vi "985x-fpga-main.vi"   [LabVIEW 2020]
uses:
  <vilib>/rvi/Emulation/niFpgaGetClockAttributes.vi
  <vilib>/rvi/Emulation/niFpgaSctlEmulationGetInTimedLoop.vi
  <vilib>/rvi/Emulation/niFpgaEmulationReportErrorSimple.vi
  <vilib>/rvi/interface/RandomDataEmulation/nirviRandomDataMultiElementFPGAFIFO.vi
  <instcachedir>/0/nirviRandomDataMultiElementFPGAFIFO_3E9965BA1FAD4E7B8DABA31768A09B1F.lvgen/nirviRandomDataMultiElementFPGAFIFO_3E9965BA1FAD4E7B8DABA31768A09B1F_001.vi
  <vilib>/rvi/interface/RandomDataEmulation/niFpgaRandomDataHandleErrors.vi
  <vilib>/rvi/eio/common/nirviEmuTemplateMethod_errors.vi
  <vilib>/rvi/Emulation/niFpgaCriticalErrorInLSC.vi
  <vilib>/rvi/DataTransferAndStorage/Container/XNode/niFpgaContainer.xnode
  <vilib>/rvi/interface/RandomDataEmulation/nirviRandomDataFpgaMultiElementTemplate.vi
  <vilib>/eio/EIONode/EIONode.xnode
  <vilib>/LabVIEW Targets/FPGA/RIO/nicrio_985x_controls.llb/CAN_IO_Frame Array U32.ctl
types:
  T1 = typedef "CAN_IO_Frame Array U32.ctl" = u32[]
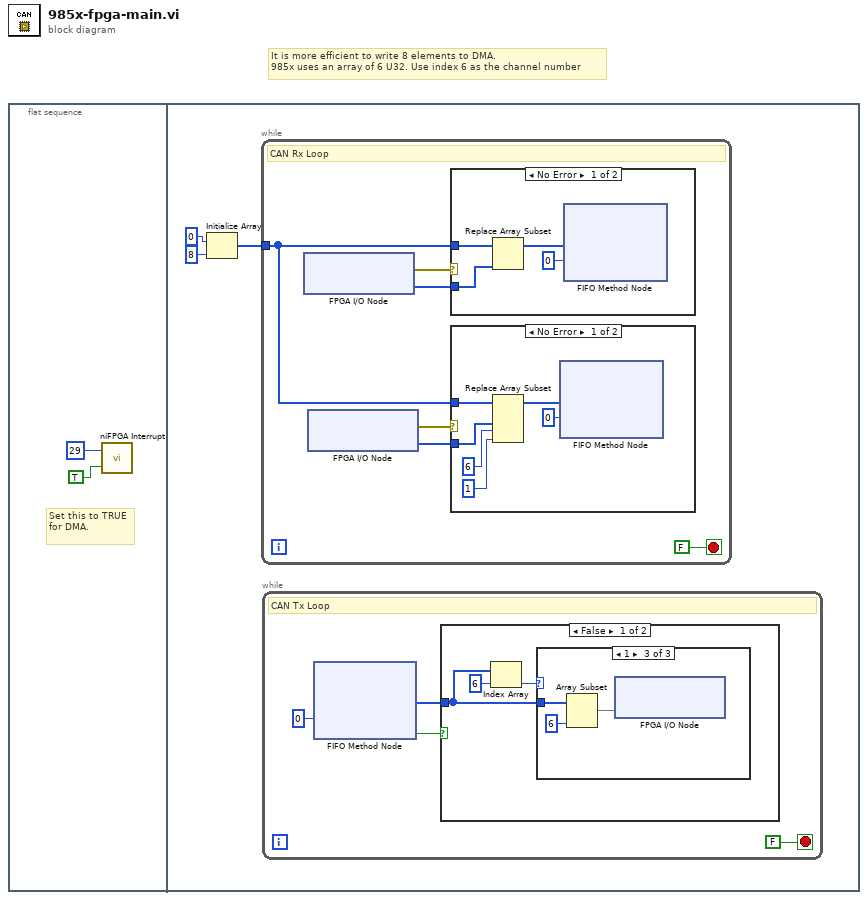
[diagram p0: block diagram]
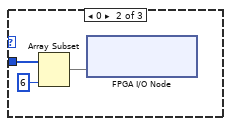
[diagram p3: hidden frame]
diagram:
  # "It is more efficient to write 8 elements to DMA.\n985x uses an array of 6 U32. Use index 6 as the channel number"
  n1 = flat-sequence {
    frame #0 {
      # "Set this to TRUE for DMA."
      n2 = call <vilib>:"niFPGA Interrupt.vi"("Wait Until Cleared (F)"=TRUE, "IRQ Number (0)"=u8 29) -> ()  [unwired: 1 in]
    }
    frame #1 {
      n3 = Initialize Array(u32 0, 8 ("dimension size")) -> (w3:u32[])
      n4 = while {
        tunnel: w3 -> [w20]
        stop <- FALSE stop-if-true
        # "CAN Rx Loop"
        n5 = xnode "FPGA I/O Node"() -> ("error out"=w24:errorcluster, "Mod8/CAN0"=w23:T1)  [unwired: 2 in, 1 out]
        n6 = xnode "FPGA I/O Node"() -> ("error out"=w22:errorcluster, "Mod8/CAN1"=w21:T1)  [unwired: 2 in, 1 out]
        n7 = case shown="No Error" w24 {
          tunnel: w20 -> [w28 _]
          tunnel: w23 -> [w27 _]
          frame No Error {
            n8 = Replace Array Subset(array=w28, new element=w27) -> (w26:u32[])  [unwired: 1 in]
            n9 = xnode ("FIFO Method Node")("Element"=w26, "Timeout"=0) -> ()  [unwired: 1 in, 2 out]
          }
          frame Error {
          }
        }
        n10 = case shown="No Error" w22 {
          tunnel: w20 -> [w34 _]
          tunnel: w21 -> [w33 _]
          frame No Error {
            n11 = Replace Array Subset(array=w34, new element #1=w33, new element #2=u32 1, index #2=6 ("index")) -> (w32:u32[])  [unwired: 1 in]
            n12 = xnode ("FIFO Method Node")("Element"=w32, "Timeout"=0) -> ()  [unwired: 1 in, 2 out]
          }
          frame Error {
          }
        }
      }
      n13 = while {
        stop <- FALSE stop-if-true
        # "CAN Tx Loop"
        n14 = xnode ("FIFO Method Node")("Timeout"=0) -> ("Element"=w7:u32[], "Timed Out?"=w8:bool)  [unwired: 1 in, 1 out]
        n15 = case shown="False" w8 {
          tunnel: w7 -> [w10 _]
          frame False {
            n16 = Index Array(array=w10, index=6) -> (element=w11:u32)
            n17 = case shown="1" w11 {
              tunnel: w10 -> [_ w15 w18]
              frame Default {
              }
              frame 0 {
                n18 = Array Subset(array=w15, length=6) -> (w13:u32[])  [unwired: 1 in]
                n19 = xnode "FPGA I/O Node"("Mod8/CAN0"=w13) -> ()  [unwired: 2 in, 2 out]
              }
              frame 1 {
                n20 = Array Subset(array=w18, length=6) -> (w16:u32[])  [unwired: 1 in]
                n21 = xnode "FPGA I/O Node"("Mod8/CAN1"=w16) -> ()  [unwired: 2 in, 2 out]
              }
            }
          }
          frame True {
          }
        }
      }
    }
  }
